vi "time_get_string.vi"(1 "utc?":bool) -> (0 "time_string":string)   [LabVIEW 2018]
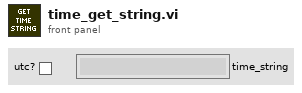
[diagram p1: front panel]
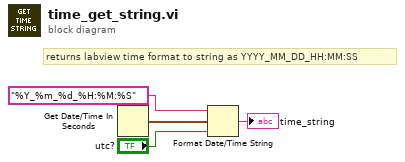
[diagram p0: block diagram]
diagram:
  # "returns labview time format to string as YYYY_MM_DD_HH:MM:SS"
  n1 = Get Date/Time In Seconds() -> (seconds since 1Jan1904=w2:timestamp)
  n2 = Format Date/Time String(time format string (%c)="%Y_%m_%d_%H:%M:%S", seconds (now)=w2, UTC format="utc?") -> (date/time string=→"time_string":string)
